vi "Write SPI.vi"(4 "CS Active Low (T)":bool=TRUE, 5 "CS Pin (None)":i32=-1, 7 "Bus":u8, 8 "error in (no error)":errorcluster, 10 "Data":string, 11 "VISA resource name in":refnum<visa-resource-name>) -> (0 "error out":errorcluster, 3 "VISA resource name":refnum<visa-resource-name>)   [LabVIEW 2023, in "CTI-Visa.lvlib"]
uses:
  CTI-Visa.lvlib
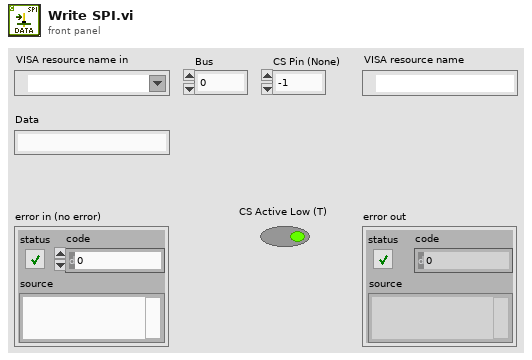
[diagram p1: front panel]
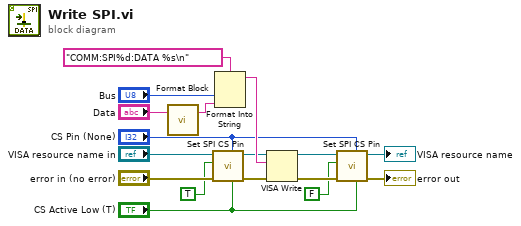
[diagram p0: block diagram]
diagram:
  n1 = call "Format Block.vi"("Data Block"="Data") -> ("Formatted Block"=w11:string)  [unwired: 6 in]
  n2 = call "Set SPI CS Pin.vi"("CS Active Low (T)"="CS Active Low (T)", "CS GPIO"="CS Pin (None)", "error in (no error)"="error in (no error)", "CS Active"=TRUE, "VISA resource name in"="VISA resource name in") -> ("error out"=w10:errorcluster, "VISA resource name"=w8:refnum<visa-resource-name>)  [unwired: 5 in]
  n3 = Format Into String(format string="COMM:SPI%d:DATA %s\n", "Bus", w11) -> (resulting string=w13:string)  [unwired: 2 in, 1 out]
  n4 = VISA Write(VISA resource name=w8, write buffer=w13, error in (no error)=w10) -> (VISA resource name out=w5:refnum<visa-resource-name>, error out=w17:errorcluster)  [unwired: 1 out]
  n5 = call "Set SPI CS Pin.vi"("CS Active Low (T)"="CS Active Low (T)", "CS GPIO"="CS Pin (None)", "error in (no error)"=w17, "CS Active"=FALSE, "VISA resource name in"=w5) -> ("error out"=→"error out":errorcluster, "VISA resource name"=→"VISA resource name":refnum<visa-resource-name>)  [unwired: 5 in]
